vi "dataset.add.path.vi"(8 "error in":errorcluster, 11 "Asset RID":string) -> (0 "error out":errorcluster, 3 "Path":string)   [LabVIEW 2020, in "asset.lvclass"]
uses:
  asset.lvclass
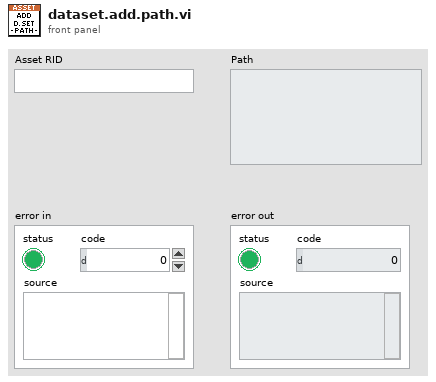
[diagram p1: front panel]
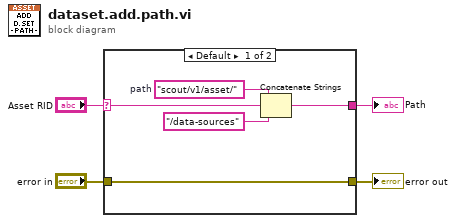
[diagram p0: block diagram]
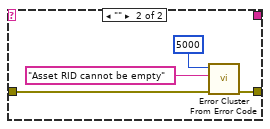
[diagram p2: hidden frame]
diagram:
  n1 = case shown="Default" "Asset RID" {
    selector: "Asset RID" -> [w7 _]
    tunnel: [w6 _] -> w3
    tunnel: "error in" -> [w5 w12]
    tunnel: [w5 w11] -> w2
    frame Default {
      w8 = "scout/v1/asset/"  # path
      n2 = Concatenate Strings(w8, w7, "/data-sources" ("string")) -> (w6:string)
    }
    frame "" {
      n3 = call <vilib>:"Error Cluster From Error Code.vi"("error in (no error)"=w12, "error message (\"\")"="Asset RID cannot be empty" ("error message (\"\")"), "error code (0)"=5000) -> ("error out"=w11:errorcluster)  [unwired: 6 in]
    }
  }
  "error out" <- w2
  "Path" <- w3
